vi "DriveModuleControl.vi"(9 "Actual State":T1={"Speed"=0.0, "Angle"={"VALUE"=0.0, "COS"=1.0, "SIN"=0.0}} {"Angle"."SIN" format="%13.4f"; "Angle"."COS" format="%13.4f"; "Angle"."VALUE" format="%13.4f"}, 10 "Desired State":T1={"Speed"=0.0, "Angle"={"VALUE"=0.0, "COS"=1.0, "SIN"=0.0}} {"Angle"."SIN" format="%13.4f"; "Angle"."COS" format="%13.4f"; "Angle"."VALUE" format="%13.4f"}, 11 "ModualNamePrefix":string) -> ()   [LabVIEW 2020]
uses:
  <vilib>/Rock Robotics/WPI/ThirdParty/JAS_Junk/TrajLib/Trajectory_Library.lvlib
  <vilib>/Rock Robotics/Network Tables/NT Write Boolean.vi
  <vilib>/Rock Robotics/Network Tables/NT Write Number.vi
  <vilib>/Rock Robotics/WPI/ThirdParty/JAS_Junk/TrajLib/TypeDef/ROTATION2D.ctl
  <vilib>/Rock Robotics/WPI/ThirdParty/JAS_Junk/TrajLib/TypeDef/SWERVE_DRIVE_MODULE_STATE.ctl
panel:
  out "error out":errorcluster
  in  "error in":errorcluster
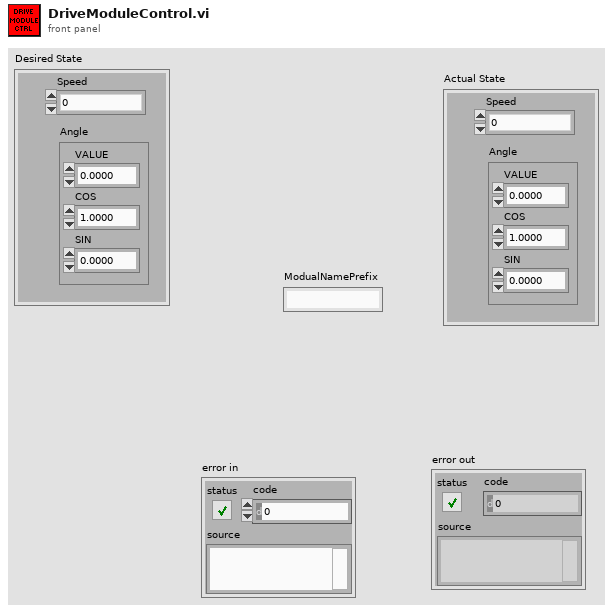
[diagram p1: front panel]
types:
  T1 = typedef "Trajectory_Library.lvlib/SWERVE_DRIVE_MODULE_STATE.ctl" = cluster{"Speed":dbl, "Angle":T2}
  T2 = typedef "Trajectory_Library.lvlib/ROTATION2D.ctl" = cluster{"VALUE":dbl, "COS":dbl, "SIN":dbl}
  T3 = typedef "WPI_MotorControlDeviceRef.ctl" = cluster{"DeviceStatus":errorcluster, "Type":T4, "PWM":cluster{"PWM Channel":T5, "DeadBand":T6}, "CAN":cluster{"Device Number":u8, "SetOutput VI Ref":variant, "GetOutput VI Ref":variant, "Enable VI Ref":variant, "Disable VI Ref":variant, "Data":variant}, "Invert":bool, "DIO PWM":cluster{"PWM \"Enable\" Channel":T5, "DIOChannel":T7, "PWM Rate":dbl}}
  T4 = typedef "WPI_MotorControlType.ctl" = enum16{"PWM", "CAN", "DIO PWM"}
  T5 = typedef "FPGA_DIOPWMChannel.ctl" = enum8{"PWM 0", "PWM 1", "PWM 2", "PWM 3", "PWM 4", "PWM 5", "PWM 6", "PWM 7", "PWM 8", "PWM 9", "PWM MXP 0", "PWM MXP 1", "PWM MXP 2", "PWM MXP 3", "PWM MXP 4", "PWM MXP 5", "PWM MXP 6", "PWM MXP 7", "PWM MXP 8", "PWM MXP 9", "Invalid"}
  T6 = typedef "WPI_PWMDeadband.ctl" = cluster{"Name":string, "maxPositivePwm":i32, "minPositivePwm":i32, "centerPwm":i32, "maxNegativePwm":i32, "minNegativePwm":i32, "angularRange":u16}
  T7 = typedef "FPGA_DIOChannel.ctl" = enum8{"DIO 0", "DIO 1", "DIO 2", "DIO 3", "DIO 4", "DIO 5", "DIO 6", "DIO 7", "DIO 8", "DIO 9", "DIO MXP 0", "DIO MXP 1", "DIO MXP 2", "DIO MXP 3", "DIO MXP 4", "DIO MXP 5", "DIO MXP 6", "DIO MXP 7", "DIO MXP 8", "DIO MXP 9", "DIO MXP 10", "DIO MXP 11", "DIO MXP 12", "DIO MXP 13", "DIO MXP 14", "DIO MXP 15", "SPI Port CS1", "SPI Port CS2", "SPI Port CS3", "SPI Port MISO", "SPI Port MOSI", "Invalid"}
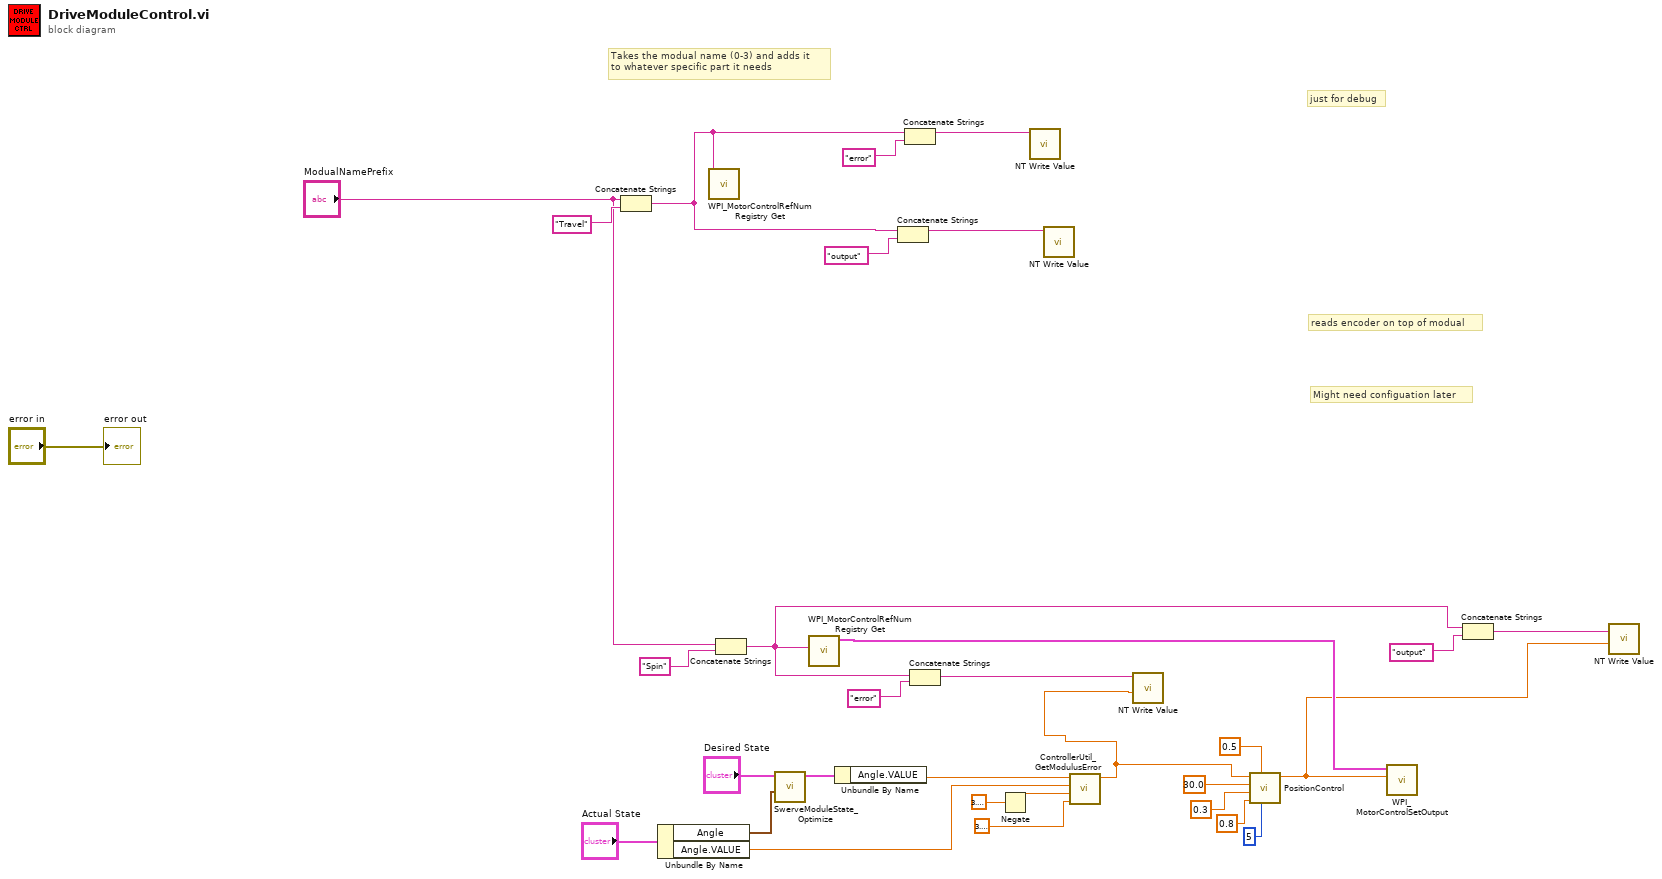
[diagram p0: block diagram]
diagram:
  # "just for debug"
  # "reads encoder on top of modual"
  # "Might need configuation later"
  # "Takes the modual name (0-3) and adds it \nto whatever specific part it needs"
  n1 = Concatenate Strings("ModualNamePrefix", "Travel" ("refnum name")) -> (w23:string)
  n2 = Unbundle By Name("Actual State") -> ("Angle"=w16:T2, "Angle.VALUE"=w12:dbl)
  n3 = call <vilib>:"WPI_MotorControlRefNum Registry Get.vi"("refnum name"=w23) -> ()  [unwired: 9 in, 2 out]
  n4 = Concatenate Strings("ModualNamePrefix", "Spin" ("refnum name")) -> (w19:string)
  n5 = call <vilib>:"SwerveModuleState_Optimize.vi"("CurrentAngle"=w16, "Desired State"="Desired State") -> ("out SWERVE_DRIVE_MODULE_STATE"=w14:T1)  [unwired: 9 in]
  n6 = call <vilib>:"WPI_MotorControlRefNum Registry Get.vi"("refnum name"=w19) -> ("MotorControlDevRef"=w5:T3)  [unwired: 9 in, 1 out]
  n7 = Unbundle By Name(w14) -> ("Angle.VALUE"=w13:dbl)
  n8 = Concatenate Strings(w23, "output" ("refnum name")) -> (w24:string)
  n9 = Concatenate Strings(w23, "error" ("refnum name")) -> (w26:string)
  n10 = Concatenate Strings(w19, "error" ("refnum name")) -> (w21:string)
  n11 = Negate(x=3.141592653589793) -> (-x=w15:dbl)
  n12 = call-poly <vilib>:"NT Write Value.vi"("name"=w26) -> ()  [unwired: 10 in, 1 out]
  n13 = call-poly <vilib>:"NT Write Value.vi"("name"=w24) -> ()  [unwired: 10 in, 1 out]
  n14 = call <vilib>:"ControllerUtil_GetModulusError.vi"("Maximum_Input"=3.141592653589793, "Minimum_Input"=w15, "Measurerment(PV)"=w12, "Reference(SP)"=w13) -> ("Error"=w2:dbl)  [unwired: 7 in]
  n15 = call-poly <vilib>:"NT Write Value.vi"("value"=w2, "name"=w21) -> ()  [unwired: 9 in, 1 out]
  n16 = call "PositionControl.vi"("ConsecutiveTargets"=5, "ErrorDeadband"=0.5, "MaxOutput"=0.8, "MinOutput"=0.3, "ErrorThreshold"=30.0, "Error"=w2) -> ("OutputValue"=w3:dbl)  [unwired: 3 in, 2 out]
  n17 = call <vilib>:"WPI_MotorControlSetOutput.vi"("Output"=w3, "MotorControlDevRef"=w5) -> ()  [unwired: 7 in, 3 out]
  n18 = Concatenate Strings(w19, "output" ("refnum name")) -> (w4:string)
  n19 = call-poly <vilib>:"NT Write Value.vi"("value"=w3, "name"=w4) -> ()  [unwired: 9 in, 1 out]
  "error out" <- "error in"
